vi "Airflow.vi"(0 "VISA resource name":refnum<visa-resource-name>, 5 "MFC Control Letter":string, 7 "Flowrate":dbl, 9 "MFC Max flowrate":dbl, 11 "error in (no error)":errorcluster) -> (4 "VISA resource name 2":refnum<visa-resource-name>, 8 "substring":string, 15 "error out":errorcluster)   [LabVIEW 2017]
panel:
  # "© The Regents of the University of California, Davis campus, 2019. This material is available as open source for research and personal use under a Creative Commons Attribution-NonCommercial-NoDerivatives 4.0 International Public License (https://creativecommons.org/licenses/by-nc-nd/4.0/)."
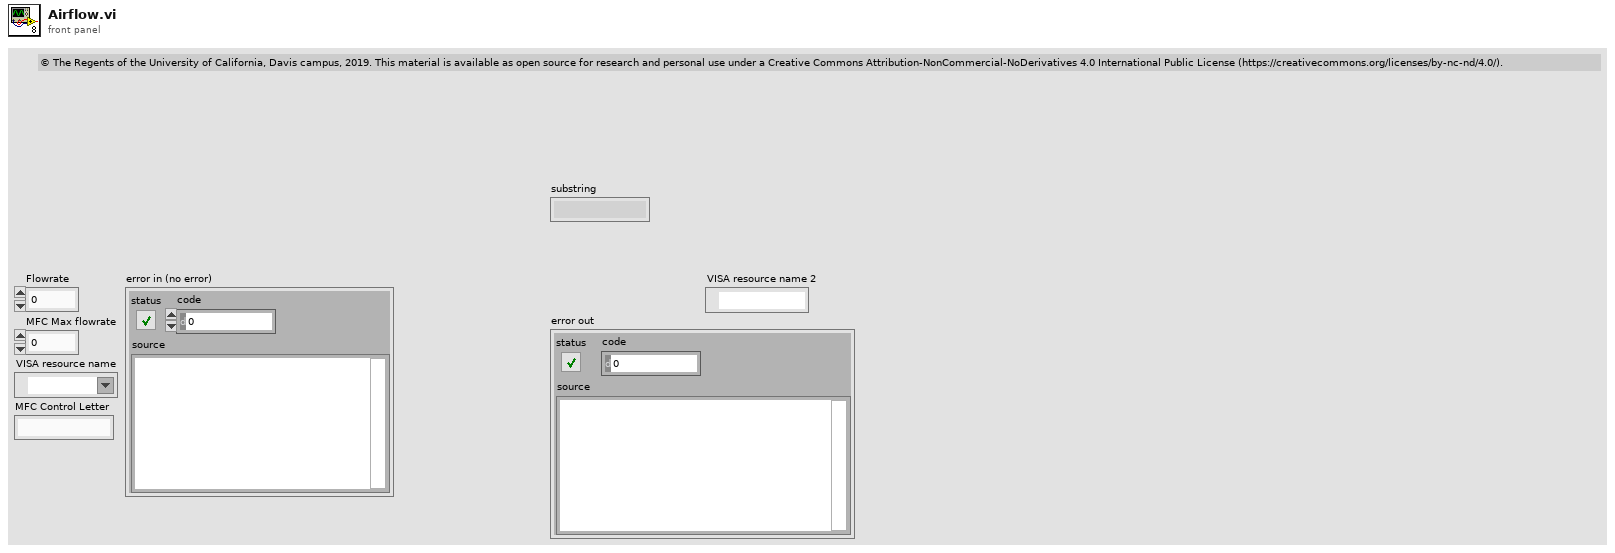
[diagram p1: front panel]
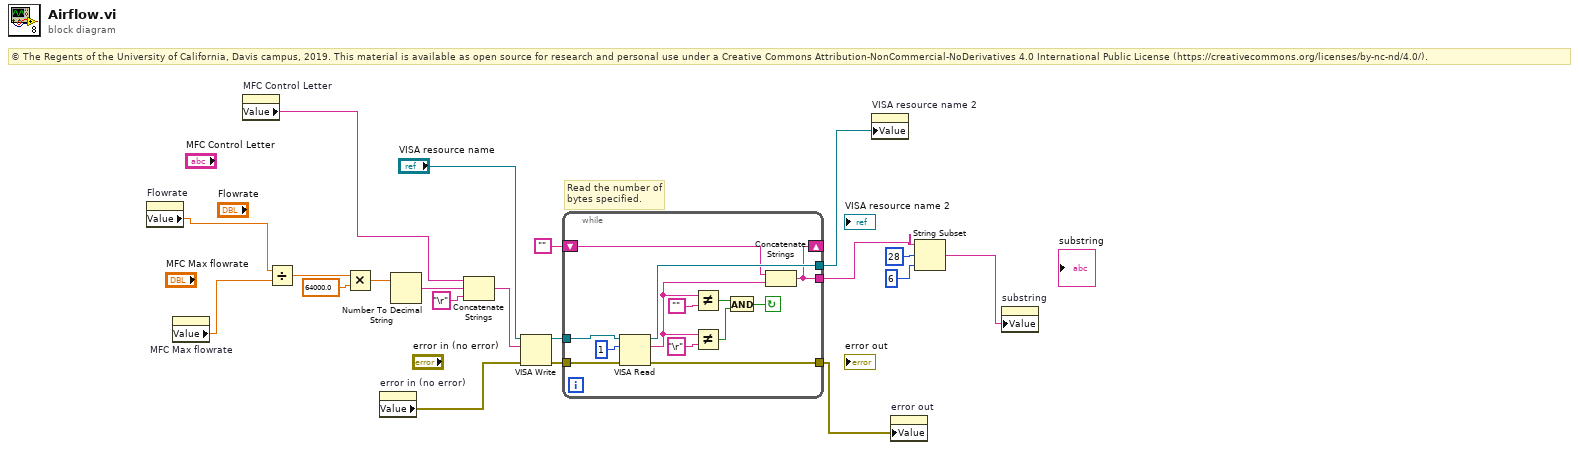
[diagram p0: block diagram]
diagram:
  # "© The Regents of the University of California, Davis campus, 2019. This material is available as open source for research and personal use under a Creative Commons Attribution-NonCommercial-NoDerivatives 4.0 International Public License (https://creativecommons.org/licenses/by-nc-nd/4.0/)."
  # "Read the number of bytes specified."
  n1 = property on="Flowrate" class="DigNum (strict)"() -> ("Value"=w6:dbl)  [unwired: 2 in, 2 out]
  n2 = property on="MFC Max flowrate" class="DigNum (strict)"() -> ("Value"=w7:dbl)  [unwired: 2 in, 2 out]
  n3 = property on="MFC Control Letter" class="Str"() -> ("Value"=w8:string)  [unwired: 2 in, 2 out]
  n4 = Divide(x=w6, y=w7) -> (x/y=w14:dbl)
  n5 = Multiply(x=w14, y=64000.0) -> (x*y=w13:dbl)
  n6 = property on="error in (no error)" class="Clust (strict)"() -> ("Value"=w3:errorcluster)  [unwired: 2 in, 2 out]
  n7 = Number To Decimal String(number=w13) -> (decimal integer string=w12:string)  [unwired: 1 in]
  n8 = Concatenate Strings(w8, w12, "\r" ("string")) -> (w20:string)
  n9 = VISA Write(VISA resource name="VISA resource name", write buffer=w20, error in (no error)=w3) -> (VISA resource name out=w19:refnum<visa-resource-name>, error out=w18:errorcluster)  [unwired: 1 out]
  n10 = while {
    tunnel: [w33] -> w4
    tunnel: [w32] -> w5
    tunnel: w18 -> [w31]
    tunnel: w19 -> [w30]
    shift-right: [w21] -> _
    shift-left: "" -> [w25]
    tunnel: [w21] -> w2
    stop <- w26 continue-if-true
    n11 = VISA Read(VISA resource name=w30, byte count=1 ("y"), error in (no error)=w31) -> (VISA resource name out=w32:refnum<visa-resource-name>, read buffer=w24:string, error out=w33:errorcluster)  [unwired: 1 out]
    n12 = Not Equal?(x=w24, y="") -> (x != y?=w29:bool)
    n13 = Not Equal?(x=w24, y="\r") -> (x != y?=w28:bool)
    n14 = And(x=w29, y=w28) -> (x .and. y?=w26:bool)
    n15 = Concatenate Strings(w25, w24) -> (w21:string)
  }
  n16 = property on="VISA resource name 2" class="VISAName"("Value"=w5) -> ()  [unwired: 2 in, 2 out]
  n17 = property on="error out" class="Clust (strict)"("Value"=w4) -> ()  [unwired: 2 in, 2 out]
  n18 = String Subset(string=w2, offset (0)=28, length (rest)=6 ("offset (0)")) -> (substring=w1:string)
  n19 = property on="substring" class="Str"("Value"=w1) -> ()  [unwired: 2 in, 2 out]
